vi "Bookout Booking.vi"(6 "Bookout List":T2[](array[typedef]) {"End Time" format="%<%d/%m/%Y\n%I:%M:%S %p>T"; "Start Time" format="%<%d/%m/%Y\n%I:%M:%S %p>T"}, 8 "error in (no error)":errorcluster, 11 "Ref In":T4={"MS SQL Connection"=refnum, "UDL File"=path "", "Time"="", "DCODE"="", "WIP+1"=0, "MC No?"=0, "POKAYOKE?"=FALSE, "Expected Result"="", "Result [Status]"="", "Clock"=0.0, "RFID"="", "WIP Queue"=refnum, "TS Parameter"={"ProfitCenterCode"="", "LineCode"="", "WorkOrderNumber"="", "Model"="", "Model_with_Prefix"="", "VendorCode"="", "SetParameterDateCode"="", "PokaYoke"=0, "Target"=1, "Live_DateCode"="", "CustomerPartNumber"="", "Hand"="", "sBarcode"=FALSE, "FCA"=0, "Ent_Stamp"=timestamp(0 s since 1904-01-01), "STS_CD"=0.0}, "Data_Queue"=[], "RFID Serial No."=""} {"TS Parameter"."FCA" format="%01d"; "TS Parameter"."Target" min=1 max=100000; "TS Parameter"."PokaYoke" min=0 max=1}) -> (0 "error out":errorcluster)   [LabVIEW 2020]
uses:
  Controls/TD SQL.ctl
  <vilib>/addons/database/Connection.llb/Conn ObjectReference.ctl
  Controls/WIP_State.ctl
  Controls/TS_Parameter.ctl
  Controls/Breakdown_List.ctl
  Controls/Loss_type.ctl
  <vilib>/Utility/error.llb/whitespace.ctl
  MS SQL/MS_Global.vi
  <vilib>/addons/database/NI_Database_API.lvlib
panel:
  out "Machine":T1(ring)
  out "Array":string[](array[string])
  out "Loss Booking In Progressing...":dbl(slide) scale=-1.0..1.0
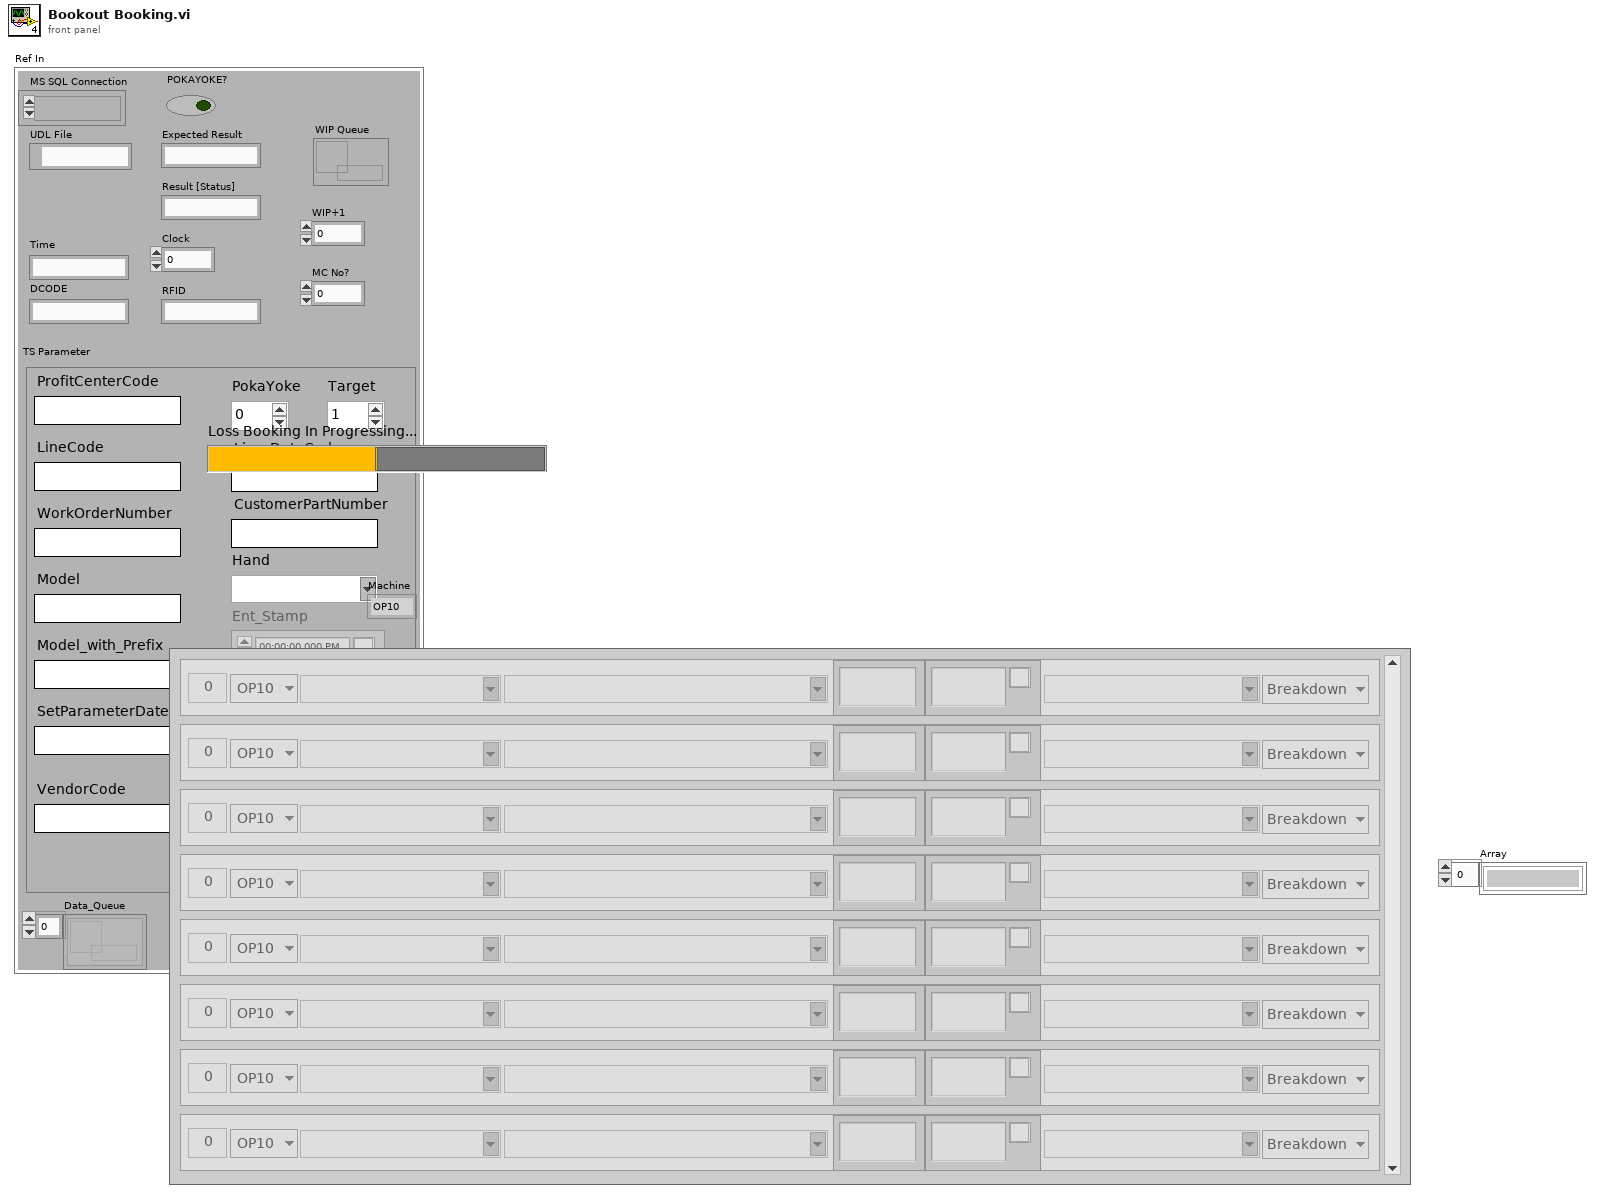
[diagram p1: front panel]
types:
  T1 = enum16{"OP10", "OP20", "OP30", "OP40", "OP50", "OP60", "OP70", "OP80", "LINE"}
  T2 = typedef "Breakdown_List.ctl" = cluster{"S.No":i32, "Reason Code":string, "Start Time":timestamp, "End Time":timestamp, "Operator":string, "Type":T3, "Machine":enum16{"OP10", "OP20", "OP30", "OP40", "OP50", "OP60", "OP70", "OP80", "LINE"}, "Reason":string}
  T3 = typedef "Loss_type.ctl" = enum16{"Breakdown", "Bookout"}
  T4 = typedef "TD SQL.ctl" = cluster{"MS SQL Connection":T5, "UDL File":path, "Time":string, "DCODE":string, "WIP+1":i64, "MC No?":i32, "POKAYOKE?":bool, "Expected Result":string, "Result [Status]":string, "Clock":dbl, "RFID":string, "WIP Queue":refnum<queue>, "TS Parameter":T6, "Data_Queue":refnum<queue>[], "RFID Serial No.":string}
  T5 = typedef "NI_Database_API.lvlib/Conn ObjectReference.ctl" = refnum<k1>
  T6 = typedef "TS_Parameter.ctl" = cluster{"ProfitCenterCode":string, "LineCode":string, "WorkOrderNumber":string, "Model":string, "Model_with_Prefix":string, "VendorCode":string, "SetParameterDateCode":string, "PokaYoke":i32, "Target":i32, "Live_DateCode":string, "CustomerPartNumber":string, "Hand":string, "sBarcode":bool, "FCA":i32, "Ent_Stamp":timestamp, "STS_CD":dbl}
  T7 = typedef "whitespace.ctl" = u16
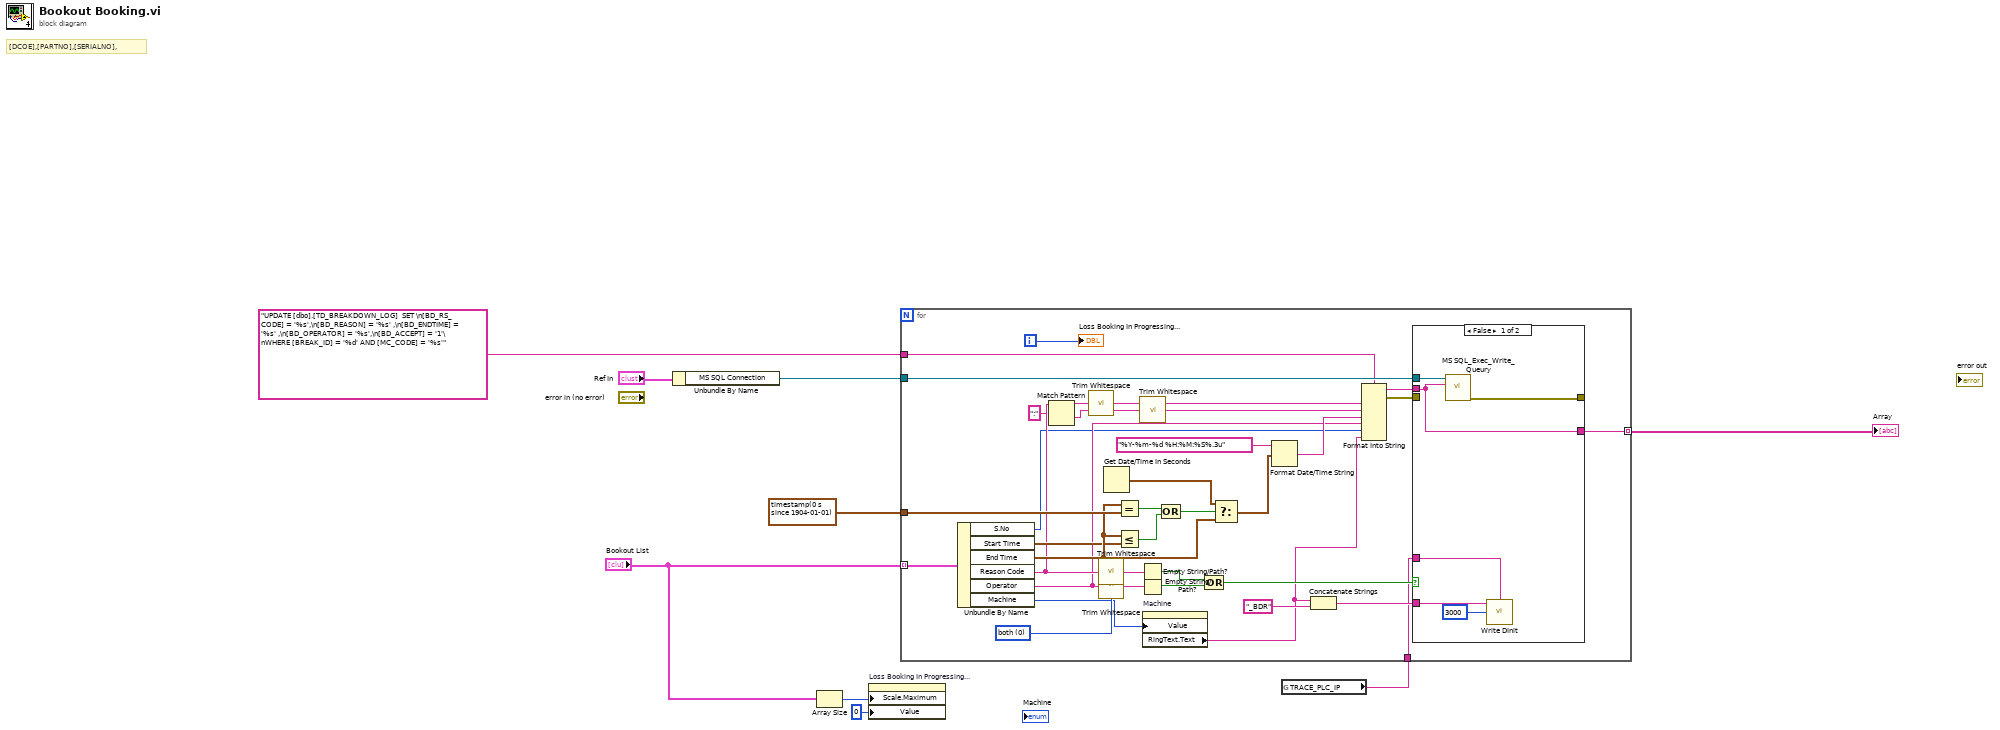
[diagram p0: block diagram]
diagram:
  # "[DCOE],[PARTNO],[SERIALNO],"
  n1 = Unbundle By Name("Ref In") -> ("MS SQL Connection"=w5:T5)
  n2 = Array Size(array="Bookout List") -> (size(s)=w3:i32)
  n3 = property on="Loss Booking In Progressing..." class="Slide (strict)"("Scale.Maximum"=w3, "Value"=u8 0 ("Delete In Process...")) -> ()  [unwired: 2 in, 2 out]
  n4 = global read "MS_Global.vi" "TRACE_PLC_IP"() -> (w1:string)
  n5 = for {
    tunnel: "Bookout List" -> [w43] mode=indexing
    tunnel: timestamp(0 s since 1904-01-01) ("Date 2") -> [w42]
    tunnel: "UPDATE [dbo].[TD_BREAKDOWN_LOG]  SET \n[BD_RS_CODE] = '%s',\n[BD_REASON] = '%s' ,\n[BD_ENDTIME] = '%s' ,\n[BD_OPERATOR] = '%s',\n[BD_ACCEPT] = '1'\nWHERE [BREAK_ID] = '%d' AND [MC_CODE] = '%s'" ("Operator") -> [w30]
    tunnel: w5 -> [w31]
    tunnel: [w16] -> w2 mode=indexing
    tunnel: w1 -> [w10]
    i -> [w17]
    w37 = T7 0 items=["both", "start of string", "end of string"] ("location (both)")
    n6 = Unbundle By Name(w43) -> ("S.No"=w20:i32, "Start Time"=w40:timestamp, "End Time"=w41:timestamp, "Reason Code"=w29:string, "Operator"=w21:string, "Machine"=w12:T1)
    n7 = Match Pattern(string=w29, regular expression=":") -> (before substring=w28:string, after substring=w15:string)  [unwired: 1 in, 2 out]
    n8 = call <vilib>:"Trim Whitespace.vi"("string"=w28) -> ("trimmed string"=w26:string)  [unwired: 1 in]
    n9 = call <vilib>:"Trim Whitespace.vi"("string"=w29, "location (both)"=w37) -> ("trimmed string"=w36:string)
    n10 = call <vilib>:"Trim Whitespace.vi"("string"=w21, "location (both)"=w37) -> ("trimmed string"=w35:string)
    n11 = Get Date/Time In Seconds() -> (seconds since 1Jan1904=w44:timestamp)
    n12 = Equal?(x=w41, y=w42) -> (x = y?=w45:bool)
    n13 = Less Or Equal?(x=w41, y=w40) -> (x <= y?=w38:bool)
    n14 = call <vilib>:"Trim Whitespace.vi"("string"=w15) -> ("trimmed string"=w25:string)  [unwired: 1 in]
    n15 = Empty String/Path?(string/path=w36) -> (empty?=w34:bool)
    n16 = Empty String/Path?(string/path=w35) -> (empty?=w33:bool)
    n17 = property on="Machine" class="Enum (strict)"("Value"=w12) -> ("RingText.Text"=w11:string)  [unwired: 2 in, 2 out]
    n18 = Compound Arithmetic op=OR(w45, w38) -> (w39:bool)
    n19 = Compound Arithmetic op=OR(w34, w33) -> (w32:bool)
    n20 = Select(t=w44, s=w39, f=w41) -> (s? t:f=w23:timestamp)
    n21 = Format Date/Time String(time format string (%c)="%Y-%m-%d %H:%M:%S%.3u", seconds (now)=w23) -> (date/time string=w22:string)  [unwired: 1 in]
    n22 = Concatenate Strings(w11, "_BDR" ("String")) -> (w13:string)
    n23 = Format Into String(format string=w30, w26, w25, w22, w21, w20, w11) -> (resulting string=w18:string, error out=w19:errorcluster)  [unwired: 2 in]
    n24 = case shown="False" w32 {
      tunnel: w31 -> [w51 _]
      tunnel: w19 -> [_ _]
      tunnel: w18 -> [w49 _]
      tunnel: [w50 _] -> _
      tunnel: [w49 _] -> w16
      tunnel: w13 -> [w47 _]
      tunnel: w10 -> [w46 _]
      frame False {
        n25 = call "MS SQL_Exec_Write_Queury.vi"("Query"=w49, "Refnum in"=w51) -> ("error out"=w50:errorcluster)  [unwired: 8 in, 1 out]
        n26 = call "Write DInit.vi"("Network Path"=w46, "Int"=3000, "Tag Name"=w47) -> ()  [unwired: 2 in]
      }
      frame True {
      }
    }
    "Loss Booking In Progressing..." <- w17
  }
  "Array" <- w2
